vi "GetLatestMeasurement.vi"(11 "Base URL":string) -> (0 "error out":errorcluster, 3 "Latest measurement":T1)   [LabVIEW 2026]
uses:
  MeasurementCluster.ctl
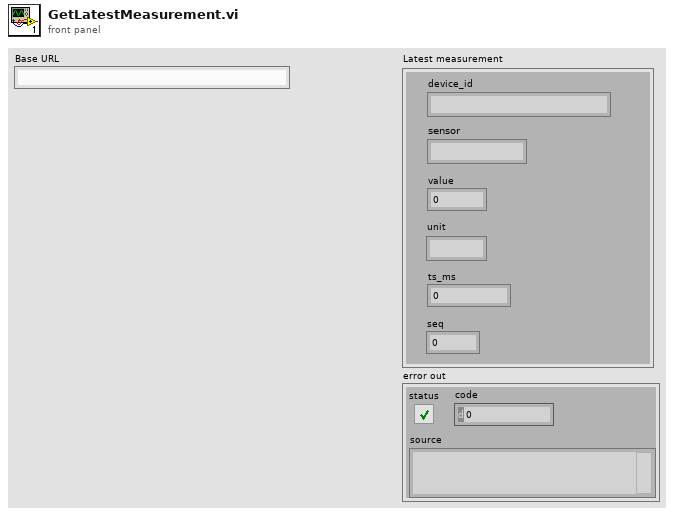
[diagram p1: front panel]
types:
  T1 = typedef "MeasurementCluster.ctl" = cluster{"device_id":string, "sensor":string, "value":dbl, "unit":string, "ts_ms":dbl, "seq":dbl}
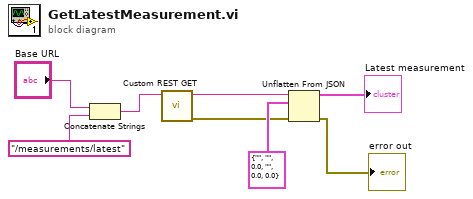
[diagram p0: block diagram]
diagram:
  n1 = Concatenate Strings("Base URL", "/measurements/latest" ("string")) -> (w7:string)
  n2 = call "Custom REST GET.vi"("Base URL"=w7) -> ("Error out"=w1:errorcluster, "body"=w6:string)  [unwired: 9 in]
  n3 = Unflatten From JSON(JSON string=w6, type and defaults=T1 {"device_id"="", "sensor"="", "value"=0.0, "unit"="", "ts_ms"=0.0, "seq"=0.0} ("Measurement"), error in (no error)=w1) -> (value=→"Latest measurement":T1, error out=→"error out":errorcluster)  [unwired: 4 in]
